vi "Read Var from Table.vi"(1 "VAR Column Index":i32=6, 2 "Current Step ID":i32, 3 "Value":string[][](array[string])) -> (0 "Numeric":dbl)   [LabVIEW 2018]
panel:
  out "error out":errorcluster
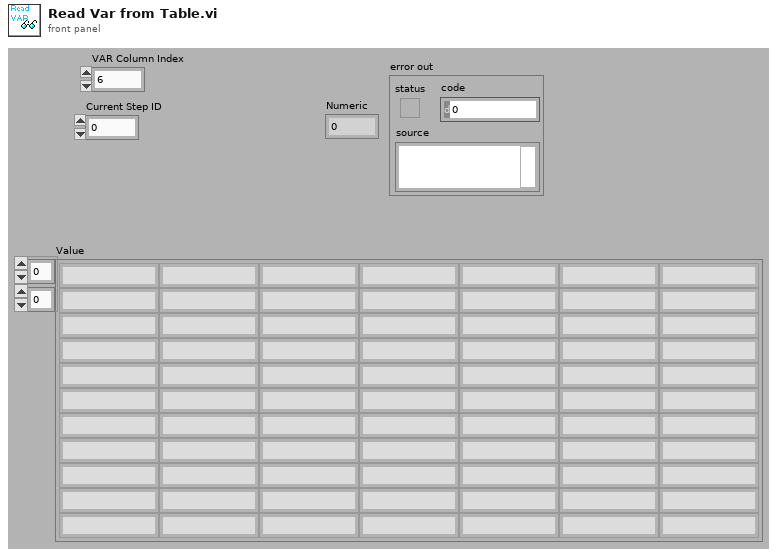
[diagram p1: front panel]
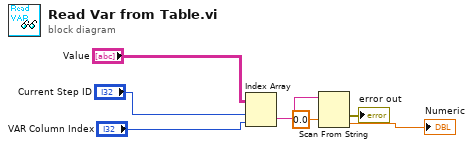
[diagram p0: block diagram]
diagram:
  n1 = Index Array(array="Value", index (row)="Current Step ID", index (col)="VAR Column Index") -> (element=w3:string)
  n2 = Scan From String(input string=w3, default 1=0.0 ("default value 1")) -> (error out=→"error out":errorcluster, output 1=→"Numeric":dbl)  [unwired: 3 in, 2 out]
